vi "LCB - DAQmx 9219 Analog Input (SubVI).vi"(0 "9219 Device Name":tag, 7 "9219 Settings":T1={"Sample Rate [Hz]"=50.0, "Number of Samples"=50, "Rolling Average"=2, "AI.ADCTimingMode"=14714} {"AI.ADCTimingMode" items=["High Resolution"=10195, "High Speed"=14712, "Best 50 Hz Rejection"=14713, "Best 60 Hz Rejection"=14714, "Custom"=10137]; "Sample Rate [Hz]" format="%#_6p"}, 11 "Error Input":errorcluster) -> (4 "9219 Signals":dbl[](array[numeric]), 15 "Analog Error":errorcluster)   [LabVIEW 2011]
uses:
  <vilib>/DAQmx/read.llb/DAQmx Read (Analog 2D DBL NChan NSamp).vi
  <vilib>/DAQmx/miscellaneous.llb/DAQmx Fill In Error Info.vi
  <vilib>/DAQmx/create/channels.llb/DAQmx Create Channel (AI-Temperature-Thermocouple).vi
  <vilib>/DAQmx/create/channels.llb/DAQmx Create Channel (AI-Current-Basic).vi
  C:/Program Files (x86)/National Instruments/LabVIEW 2011/resource/objmgr/daqmx.rc
panel:
  out "Available Samples per Channel":u32
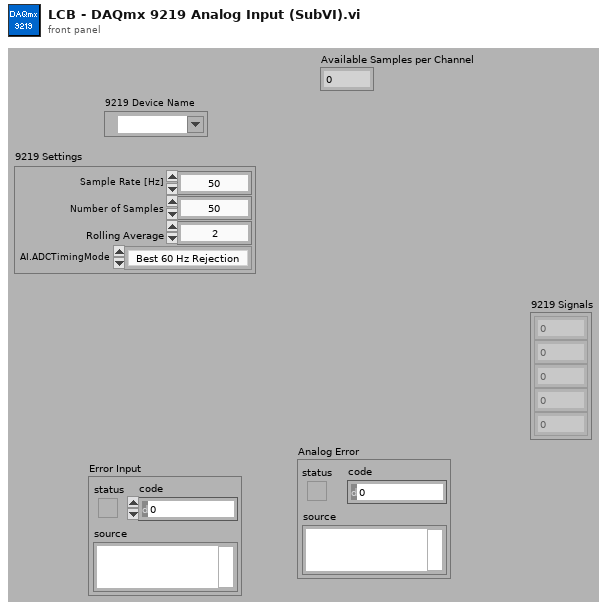
[diagram p1: front panel]
types:
  T1 = cluster{"Sample Rate [Hz]":dbl, "Number of Samples":i32, "Rolling Average":i32, "AI.ADCTimingMode":i32}
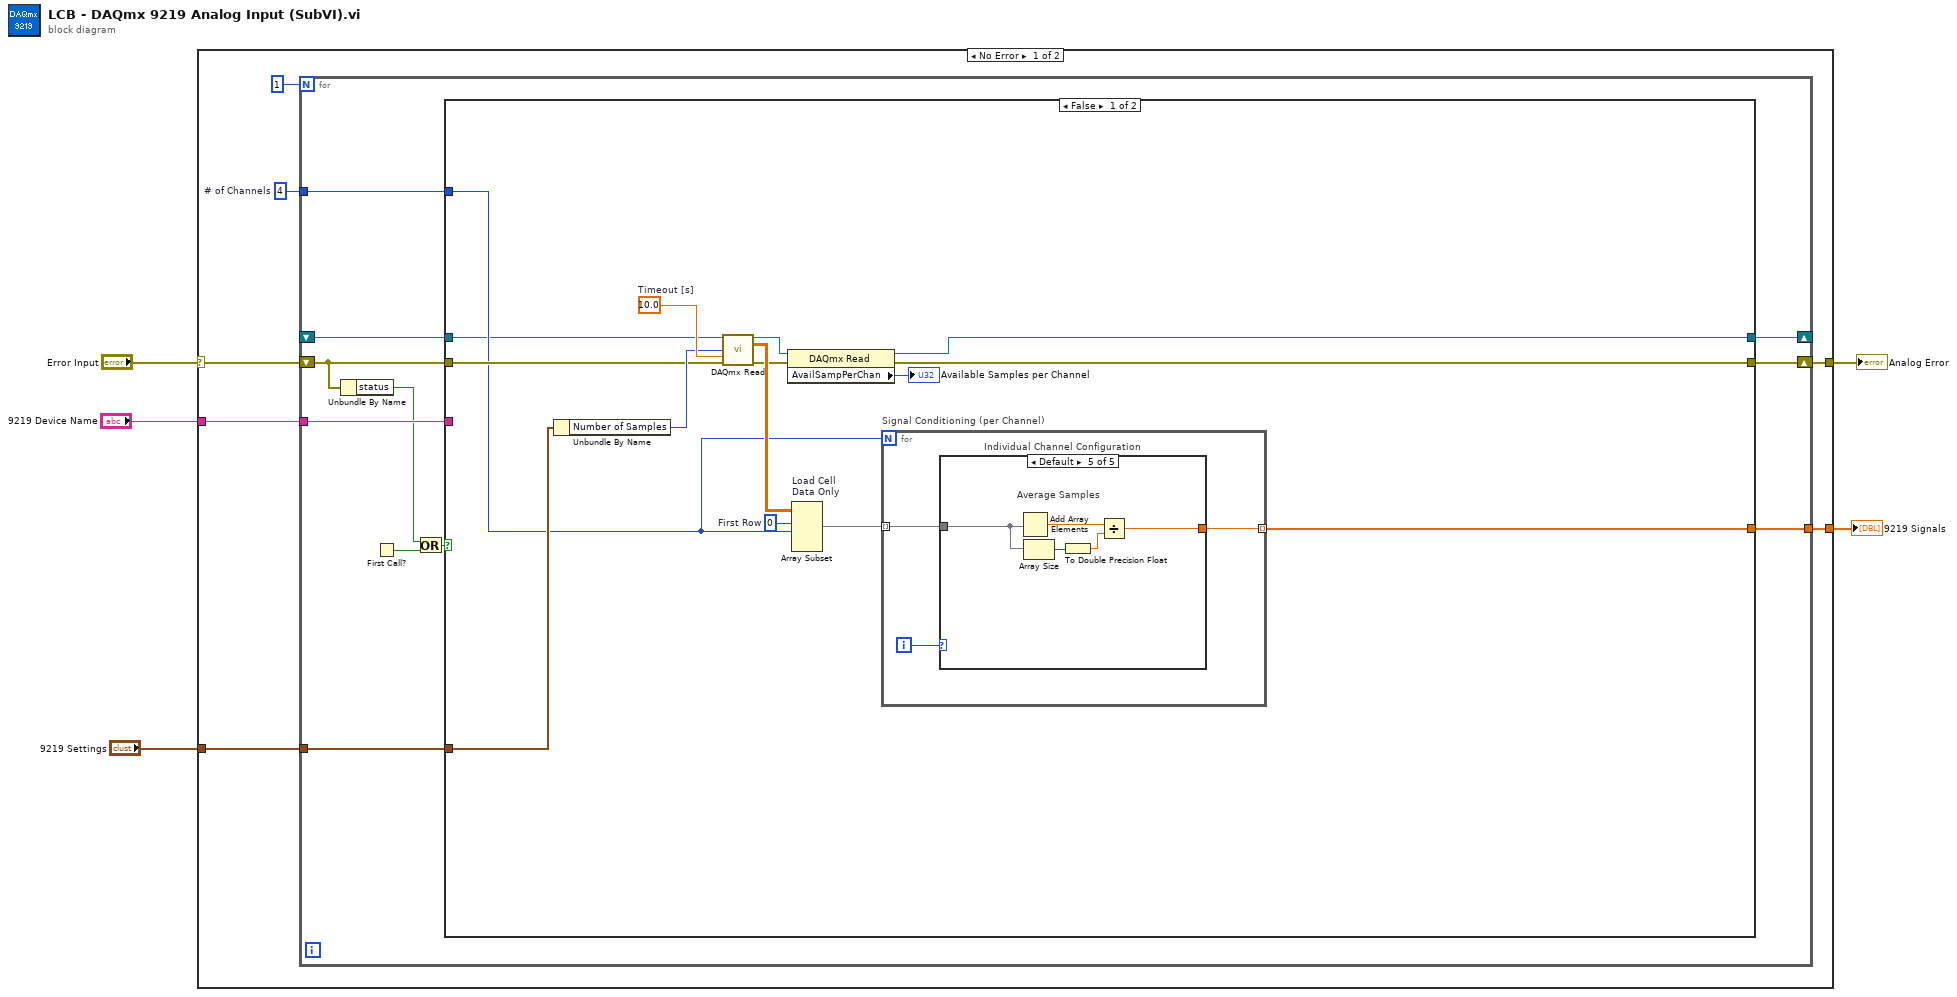
[diagram p0: block diagram]
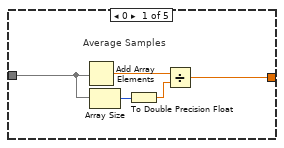
[diagram p2: hidden frame]
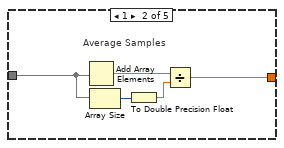
[diagram p3: hidden frame]
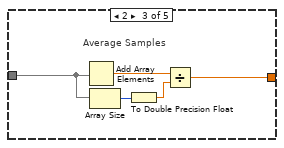
[diagram p4: hidden frame]
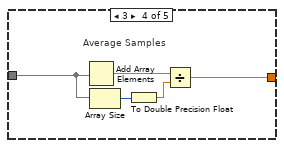
[diagram p5: hidden frame]
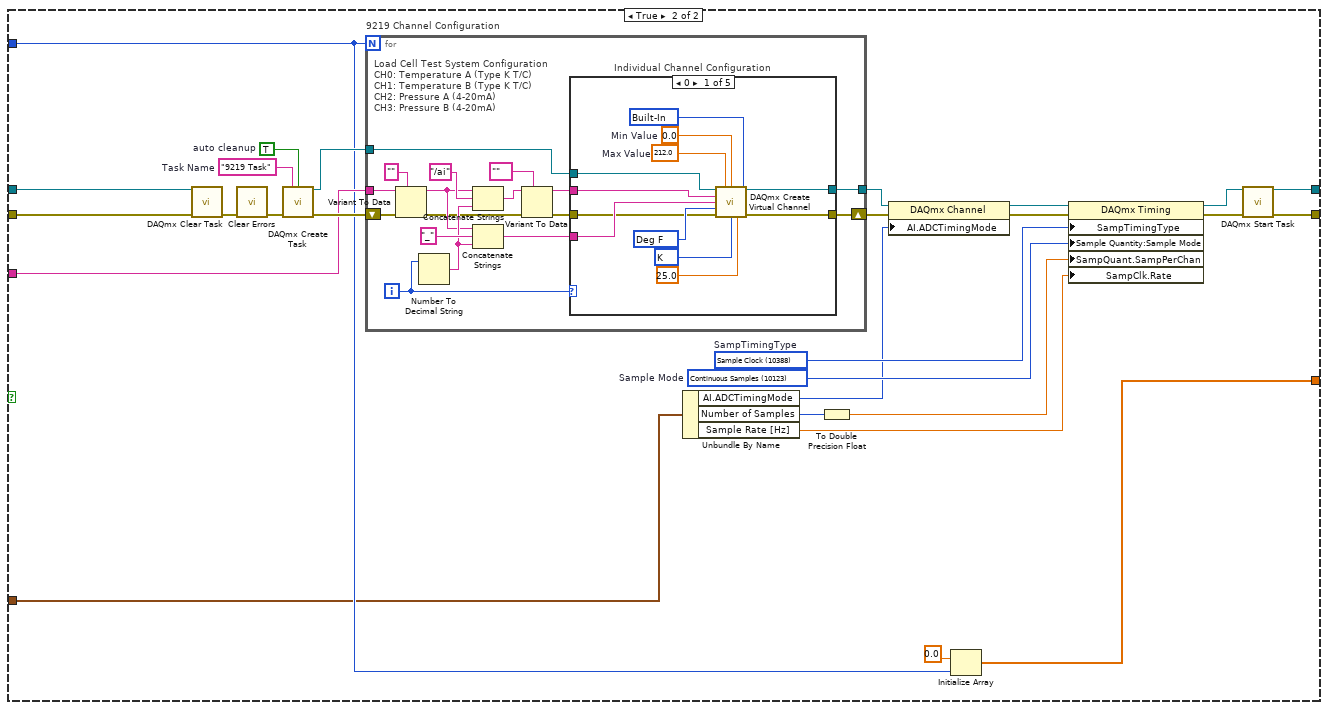
[diagram p6: hidden frame]
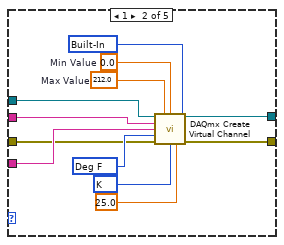
[diagram p7: hidden frame]
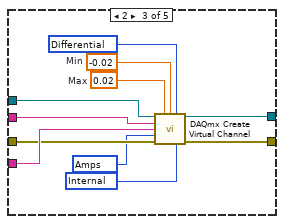
[diagram p8: hidden frame]
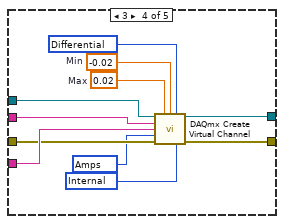
[diagram p9: hidden frame]
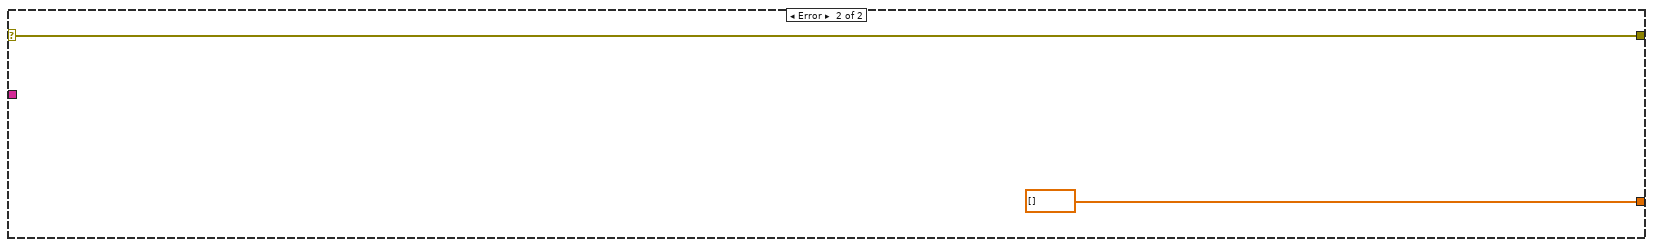
[diagram p11: hidden frame]
diagram:
  n1 = case shown="No Error" "Error Input" {
    selector: "Error Input" -> [w6 w160]
    tunnel: [w12 dbl[] []] -> w5
    tunnel: [w11 w160] -> w4
    tunnel: "9219 Settings" -> [w10 _]
    tunnel: "9219 Device Name" -> [w8 _]
    frame No Error {
      w7 = 4  # # of Channels
      n2 = for {
        N: 1 -> [_]
        shift-right: [w23] -> _
        shift-left: _ -> [w21]
        shift-right: [w22] -> w11
        shift-left: w6 -> [w20]
        tunnel: w10 -> [w18]
        tunnel: [w17] -> w12
        tunnel: w8 -> [w16]
        tunnel: w7 -> [w13]
        n3 = Unbundle By Name(w20) -> ("status"=w14:bool)
        n4 = First Call?() -> (First Call?: T/F=w15:bool)
        n5 = Or(x=w14, y=w15) -> (x .or. y?=w19:bool)
        n6 = case shown="False" w19 {
          tunnel: [w25 w87] -> w23
          tunnel: [w27 w86] -> w22
          tunnel: w20 -> [w32 w93]
          tunnel: w21 -> [w29 w92]
          tunnel: w18 -> [w34 w74]
          tunnel: [w30 w84] -> w17
          tunnel: w16 -> [_ w82]
          tunnel: w13 -> [w31 w78]
          frame False {
            w37 = 0  # First Row
            w38 = 10.0  # Timeout [s]
            n7 = Unbundle By Name(w34) -> ("Number of Samples"=w33:i32)
            n8 = call-poly <vilib>:"DAQmx Read.vi"("task/channels in"=w29, "number of samples per channel"=w33, "timeout"=w38, "error in"=w32) -> ("task out"=w26:refnum<k21>, "data"=w36:dbl[][], "error out"=w28:errorcluster)  [unwired: 9 in]
            n9 = property class="DAQmx Read"(reference=w26, error in=w28) -> (reference out=w25:refnum<k21>, error out=w27:errorcluster, "AvailSampPerChan"=→"Available Samples per Channel":u32)
            n10 = Array Subset "Load Cell\nData Only"(array=w36, index (row)=w37, length (row)=w31) -> (w35:dbl[][])  [unwired: 2 in]
            n11 = for "Signal Conditioning (per Channel)" {
              N: w31 -> [_]
              tunnel: w35 -> [w40] mode=indexing
              tunnel: [w39] -> w30 mode=indexing
              i -> [w41]
              n12 = case "Individual Channel Configuration" shown="Default" w41 {
                tunnel: w40 -> [w43 w48 w53 w58 w63]
                tunnel: [w42 w47 w52 w57 w62] -> w39
                frame 0 {
                  # "Average Samples"
                  n13 = Add Array Elements(numeric array=w43) -> (sum=w44:dbl)
                  n14 = Array Size(array=w43) -> (size(s)=w45:i32)
                  n15 = To Double Precision Float(number=w45) -> (double precision float=w46:dbl)
                  n16 = Divide(x=w44, y=w46) -> (x/y=w42:dbl)
                }
                frame 1 {
                  # "Average Samples"
                  n17 = Add Array Elements(numeric array=w48) -> (sum=w49:dbl)
                  n18 = Array Size(array=w48) -> (size(s)=w50:i32)
                  n19 = To Double Precision Float(number=w50) -> (double precision float=w51:dbl)
                  n20 = Divide(x=w49, y=w51) -> (x/y=w47:dbl)
                }
                frame 2 {
                  # "Average Samples"
                  n21 = Add Array Elements(numeric array=w53) -> (sum=w54:dbl)
                  n22 = Array Size(array=w53) -> (size(s)=w55:i32)
                  n23 = To Double Precision Float(number=w55) -> (double precision float=w56:dbl)
                  n24 = Divide(x=w54, y=w56) -> (x/y=w52:dbl)
                }
                frame 3 {
                  # "Average Samples"
                  n25 = Add Array Elements(numeric array=w58) -> (sum=w59:dbl)
                  n26 = Array Size(array=w58) -> (size(s)=w60:i32)
                  n27 = To Double Precision Float(number=w60) -> (double precision float=w61:dbl)
                  n28 = Divide(x=w59, y=w61) -> (x/y=w57:dbl)
                }
                frame Default {
                  # "Average Samples"
                  n29 = Add Array Elements(numeric array=w63) -> (sum=w64:dbl)
                  n30 = Array Size(array=w63) -> (size(s)=w65:i32)
                  n31 = To Double Precision Float(number=w65) -> (double precision float=w66:dbl)
                  n32 = Divide(x=w64, y=w66) -> (x/y=w62:dbl)
                }
              }
            }
          }
          frame True {
            w75 = 10123 items=["Finite Samples"=10178, "Continuous Samples"=10123, "Hardware Timed Single Point"=12522]  # Sample Mode
            w76 = 10388 items=["Sample Clock"=10388, "Burst Handshake"=12548, "Handshake"=10389, "Implicit"=10451, "On Demand"=10390, "Change Detection"=12504, "Pipelined Sample Clock"=14668]  # SampTimingType
            w91 = "9219 Task"  # Task Name
            w90 = TRUE  # auto cleanup
            n33 = call <vilib>:"DAQmx Clear Task.vi"("task in"=w92, "error in"=w93) -> ("error out"=w89:errorcluster)  [unwired: 13 in]
            n34 = call <vilib>:"Clear Errors.vi"("error in (no error)"=w89) -> ("error out"=w88:errorcluster)  [unwired: 6 in]
            n35 = call <vilib>:"DAQmx Create Task.vi"("new task name"=w91, "auto cleanup"=w90, "error in"=w88) -> ("task out"=w81:refnum<k21>, "error out"=w83:errorcluster)  [unwired: 11 in]
            n36 = for "9219 Channel Configuration" {
              N: w78 -> [_]
              tunnel: w81 -> [w110]
              tunnel: [w109] -> w80
              shift-right: [w108] -> w79
              shift-left: w83 -> [w94]
              tunnel: w82 -> [w98]
              i -> [w97]
              # "Load Cell Test System Configuration\nCH0: Temperature A (Type K T/C)\nCH1: Temperature B (Type K T/C)\nCH2: Pressure A (4-20mA)\nCH3: Pressure B (4-20mA)"
              n37 = Variant To Data(error in=w94, type="" ("channel name"), Variant=w98) -> (data=w99:string, error out=w95:errorcluster)
              n38 = Number To Decimal String(number=w97) -> (decimal integer string=w105:string)  [unwired: 1 in]
              n39 = Concatenate Strings(w99, "/ai" ("channel name"), w105) -> (w102:string)
              n40 = Concatenate Strings(w99, "_" ("channel name"), w105) -> (w101:string)
              n41 = Variant To Data(error in=w95, type=tag "" ("physical channels"), Variant=w102) -> (data=w103:tag, error out=w96:errorcluster)
              n42 = case "Individual Channel Configuration" shown="0" w97 {
                tunnel: w110 -> [w122 w134 w145 w156 w157]
                tunnel: w96 -> [w118 w130 w142 w153 w158]
                tunnel: [w112 w124 w141 w152 w157] -> w109
                tunnel: [w111 w123 w140 w151 w158] -> w108
                tunnel: w103 -> [w121 w133 w144 w155 _]
                tunnel: w101 -> [w120 w132 w143 w154 _]
                frame 0 {
                  w113 = 10200 items=["Built-In"=10200, "Constant Value"=10116, "Channel"=10113] ("cjc source")
                  w115 = 10073 items=["J"=10072, "K"=10073, "N"=10077, "R"=10082, "S"=10085, "T"=10086, "B"=10047, "E"=10055] ("thermocouple type")
                  w116 = 0.0  # Min Value
                  w117 = 212.0  # Max Value
                  w119 = 10144 items=["Deg C"=10143, "Deg F"=10144, "Kelvins"=10325, "Deg R"=10145, "From Custom Scale"=10065] ("units")
                  n43 = call-poly <vilib>:"DAQmx Create Virtual Channel.vi"("task in"=w122, "maximum value"=w117, "minimum value"=w116, "physical channels"=w121, "cjc source"=w113, "name to assign"=w120, "units"=w119, "error in"=w118, "thermocouple type"=w115, "cjc value"=25.0) -> ("task out"=w112:refnum<k21>, "error out"=w111:errorcluster)  [unwired: 4 in]
                }
                frame 1 {
                  w125 = 10200 items=["Built-In"=10200, "Constant Value"=10116, "Channel"=10113] ("cjc source")
                  w127 = 10073 items=["J"=10072, "K"=10073, "N"=10077, "R"=10082, "S"=10085, "T"=10086, "B"=10047, "E"=10055] ("thermocouple type")
                  w128 = 0.0  # Min Value
                  w129 = 212.0  # Max Value
                  w131 = 10144 items=["Deg C"=10143, "Deg F"=10144, "Kelvins"=10325, "Deg R"=10145, "From Custom Scale"=10065] ("units")
                  n44 = call-poly <vilib>:"DAQmx Create Virtual Channel.vi"("task in"=w134, "maximum value"=w129, "minimum value"=w128, "physical channels"=w133, "cjc source"=w125, "name to assign"=w132, "units"=w131, "error in"=w130, "thermocouple type"=w127, "cjc value"=25.0) -> ("task out"=w124:refnum<k21>, "error out"=w123:errorcluster)  [unwired: 4 in]
                }
                frame 2 {
                  w135 = 10342 items=["Amps"=10342, "From Custom Scale"=10065] ("units")
                  w136 = -0.02  # Min
                  w137 = 0.02  # Max
                  w138 = 10106 items=["default"=-1, "RSE"=10083, "NRSE"=10078, "Differential"=10106, "Pseudodifferential"=12529] ("input terminal configuration")
                  w139 = 10200 items=["default"=-1, "Internal"=10200, "External"=10167] ("shunt resistor location")
                  n45 = call-poly <vilib>:"DAQmx Create Virtual Channel.vi"("task in"=w145, "maximum value"=w137, "minimum value"=w136, "input terminal configuration"=w138, "physical channels"=w144, "name to assign"=w143, "units"=w135, "error in"=w142, "shunt resistor location"=w139) -> ("task out"=w141:refnum<k21>, "error out"=w140:errorcluster)  [unwired: 5 in]
                }
                frame 3 {
                  w146 = 10342 items=["Amps"=10342, "From Custom Scale"=10065] ("units")
                  w147 = -0.02  # Min
                  w148 = 0.02  # Max
                  w149 = 10106 items=["default"=-1, "RSE"=10083, "NRSE"=10078, "Differential"=10106, "Pseudodifferential"=12529] ("input terminal configuration")
                  w150 = 10200 items=["default"=-1, "Internal"=10200, "External"=10167] ("shunt resistor location")
                  n46 = call-poly <vilib>:"DAQmx Create Virtual Channel.vi"("task in"=w156, "maximum value"=w148, "minimum value"=w147, "input terminal configuration"=w149, "physical channels"=w155, "name to assign"=w154, "units"=w146, "error in"=w153, "shunt resistor location"=w150) -> ("task out"=w152:refnum<k21>, "error out"=w151:errorcluster)  [unwired: 5 in]
                }
                frame Default {
                }
              }
            }
            n47 = Unbundle By Name(w74) -> ("AI.ADCTimingMode"=w67:i32, "Number of Samples"=w73:i32, "Sample Rate [Hz]"=w71:dbl)
            n48 = To Double Precision Float(number=w73) -> (double precision float=w72:dbl)
            n49 = property class="DAQmx Channel"(reference=w80, error in=w79, "AI.ADCTimingMode"=w67) -> (reference out=w77:refnum<k21>, error out=w70:errorcluster)
            n50 = Initialize Array(0.0, w78) -> (w84:dbl[])
            n51 = property class="DAQmx Timing"(reference=w77, error in=w70, "SampTimingType"=w76, "Sample Quantity:Sample Mode"=w75, "SampQuant.SampPerChan"=w72, "SampClk.Rate"=w71) -> (reference out=w69:refnum<k21>, error out=w68:errorcluster)
            n52 = call <vilib>:"DAQmx Start Task.vi"("task/channels in"=w69, "error in"=w68) -> ("task out"=w87:refnum<k21>, "error out"=w86:errorcluster)  [unwired: 12 in]
          }
        }
      }
    }
    frame Error {
    }
  }
  "9219 Signals" <- w5
  "Analog Error" <- w4
